vi "XLP80_CAN_MaskBytes_Test01.vi"() -> ()   [LabVIEW 2021]
uses:
  XLP80_FGlob/1886_FGlob_TDefs_Enum_FGlobItems.ctl
  XLP80_Globals/Globals_Settings_XLP80.vi
panel:
  out "Data OUT":u8[](array[numeric])=[0, 7, 255, 248, 0, 24, 0, 0] format="%.0x"
  out "Boolean array Out":bool[](array[boolean])=[FALSE, FALSE, FALSE, FALSE, FALSE, FALSE, FALSE, FALSE, TRUE, TRUE, TRUE, FALSE, FALSE, FALSE, FALSE, FALSE, TRUE, TRUE, TRUE, TRUE, TRUE, TRUE, TRUE, TRUE, FALSE, FALSE, FALSE, TRUE, TRUE, TRUE, TRUE, TRUE, FALSE, FALSE, FALSE, FALSE, FALSE, FALSE, FALSE, FALSE, FALSE, FALSE, FALSE, TRUE, TRUE, FALSE, FALSE, FALSE, FALSE, FALSE, FALSE, FALSE, FALSE, FALSE, FALSE, FALSE, FALSE, FALSE, FALSE, FALSE, FALSE, FALSE, FALSE, FALSE]
  in  "AO Values IN 2":dbl[](array[numeric])=[65535.0, 3.0] format="%.6f"
  in  "Signal Name Write 2":string[](array[string])=["Signal1", "Signal2"]
  out "err out":errorcluster caption="error"
  out "AI Values OUT":dbl[](array[numeric])=[33882.882] format="%.6f"
  in  "stop":bool
  in  "PEAK CANData Read":T1(array[cluster])=[{"ID"=1281, "MSG type"=enum."STD", "LEN"=8, "DATA"=[0, 0, 0, 0, 2, 3, 5, 2]}] {"DATA" format="%.0x"; "ID" format="%.0x"}
  in  "AO Values IN":dbl[](array[numeric])=[1.2, 2.2, 15.0, 14.0] format="%.6f"
  out "CANData Write":T1(array[cluster])=[{"ID"=2047, "MSG type"=enum."STD", "LEN"=8, "DATA"=[0, 7, 255, 248, 0, 24, 0, 0]}] {"DATA" format="%.0x"; "ID" format="%.0x"}
  in  "DBC":path=path "G:/07_GLOBE/00_git/XLP80/02_Documentation/Daten Albert_10-08-2022/TestDBC.dbc"
  in  "Signal Name Write":string[](array[string])=["C07_BAT_s_Max_Cell_Voltage", "C07_BAT_s_Min_Cell_Voltage", "C07_BAT_s_Max_Cell_Temperature", "C07_BAT_s_Min_Cell_Temperature"]
  in  "Signal Name Read":string[](array[string])=["C07_BAT_s_Battery_Voltage"]
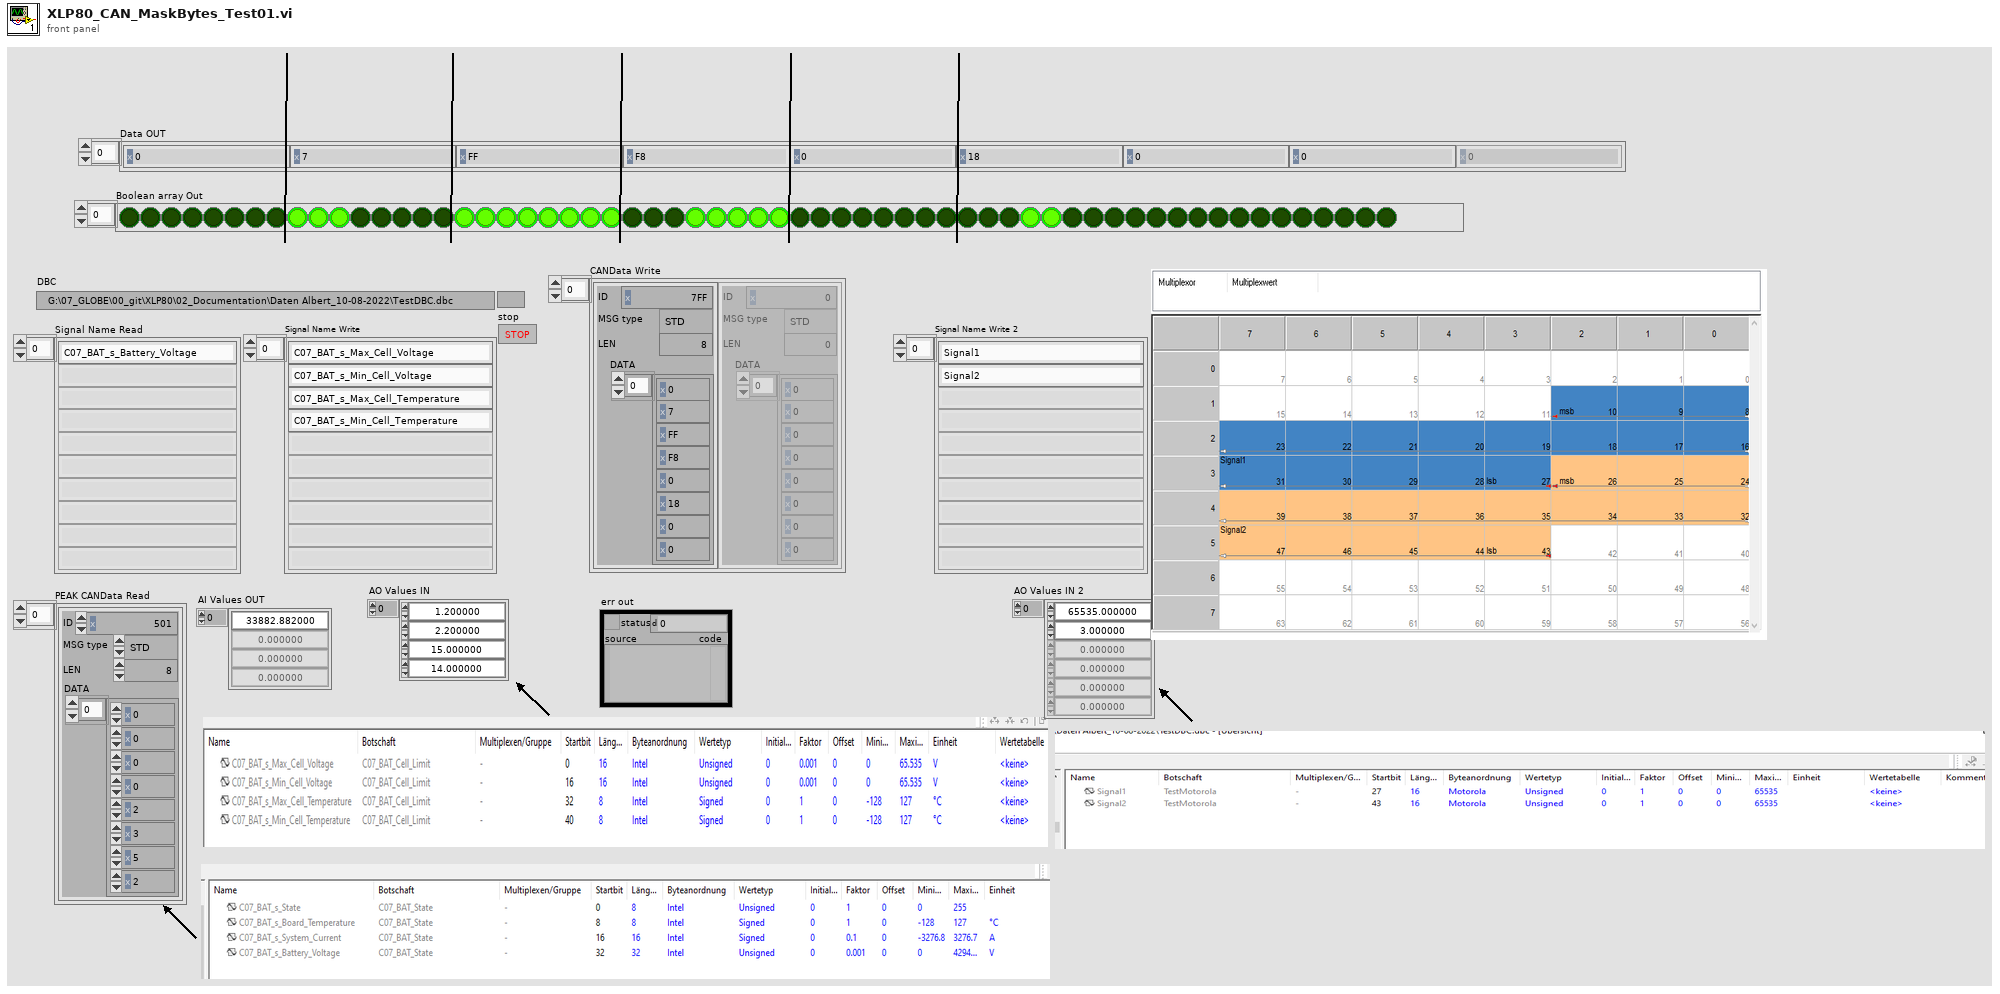
[diagram p1: front panel]
types:
  T1 = cluster{"ID":u32, "MSG type":enum8{"STD", "RTR", "XTD", "XTD RTR", "STATUS"}, "LEN":i8, "DATA":u8[]}[]
  T2 = typedef "1886_FGlob_TDefs_Enum_FGlobItems.ctl" = enum16{"Put one", "Put all", "Recall one", "Recall all"}
  T3 = cluster{"DBC":path, "Signal Name Read":string[], "Signal Name Write 2":string[]}
  T4 = typedef "PCANBasic.lvlib/CAN MSG Cluster.ctl" = cluster{"ID":u32, "MSG type":enum8{"STD", "RTR", "XTD", "XTD RTR", "STATUS"}, "LEN":i8, "DATA":u8[]}
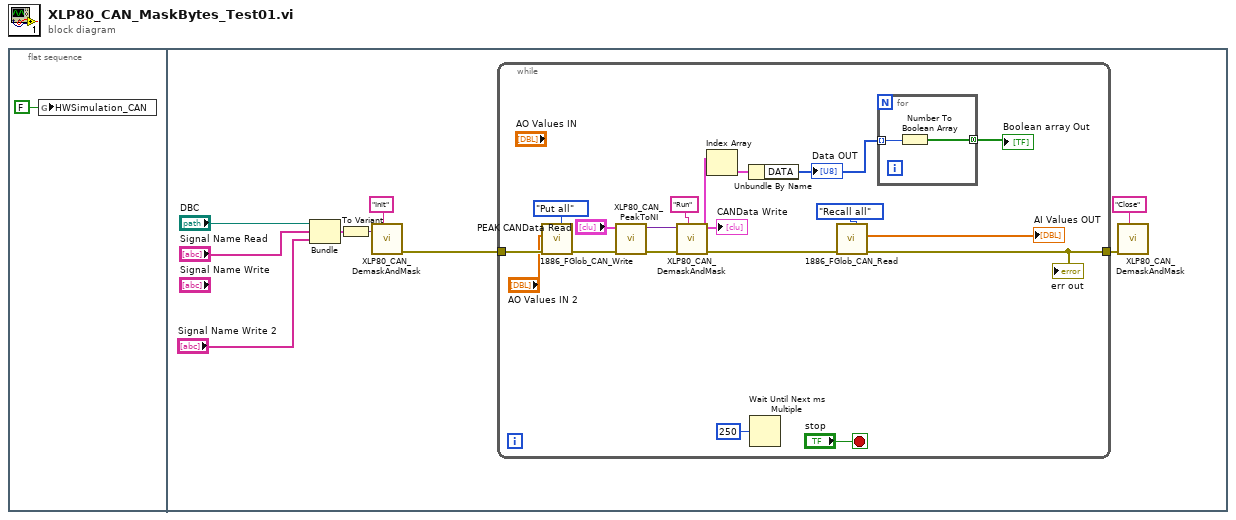
[diagram p0: block diagram]
diagram:
  n1 = flat-sequence {
    frame #0 {
      n2 = global write "Globals_Settings_XLP80.vi" "HWSimulation_CAN"(FALSE ("HWSimulation_CAN")) -> ()
    }
    frame #1 {
      n3 = Bundle("DBC"="DBC", "Signal Name Read"="Signal Name Read", "Signal Name Write 2"="Signal Name Write 2") -> (w10:T3)  [unwired: 1 in]
      n4 = To Variant(anything=w10) -> (Variant=w7:variant)
      n5 = call "XLP80_CAN_DemaskAndMask.vi"("Function"="Init", "Variant"=w7) -> ("error out"=w3:errorcluster)  [unwired: 8 in, 1 out]
      n6 = while {
        tunnel: w3 -> [w26]
        tunnel: [w18] -> w4
        stop <- "stop" stop-if-true
        n7 = call "1886_FGlob_CAN_Write.vi"("Function (Recall One)"=1886_FGlob_TDefs_Enum_FGlobItems."Put all", "AO Values IN"="AO Values IN 2") -> ()  [unwired: 7 in, 3 out]
        n8 = call "XLP80_CAN_PeakToNI.vi"("error in"=w26, "PEAK CANData Read"="PEAK CANData Read") -> ("error out"=w25:errorcluster, "NI Data OUT"=w24:variant)  [unwired: 8 in]
        n9 = call "XLP80_CAN_DemaskAndMask.vi"("Function"="Run", "err in"=w25, "Variant"=w24) -> ("error out"=w19:errorcluster, "CANData Write"=w14:T4[])  [unwired: 7 in]
        "CANData Write" <- w14
        n10 = Index Array(array=w14) -> (element=w13:T4)  [unwired: 1 in]
        n11 = Unbundle By Name(w13) -> ("DATA"=w12:u8[])
        "Data OUT" <- w12
        n12 = Wait Until Next ms Multiple(millisecond multiple=u32 250) -> ()  [unwired: 1 out]
        n13 = call "1886_FGlob_CAN_Read.vi"("Function (Recall One)"=1886_FGlob_TDefs_Enum_FGlobItems."Recall all", "err in"=w19) -> ("err out"=w18:errorcluster, "AI Values OUT"=→"AI Values OUT":dbl[])  [unwired: 7 in, 1 out]
        "err out" <- w18
        n14 = for {
          tunnel: w12 -> [w29] mode=indexing
          tunnel: [w28] -> w11 mode=concatenating
          n15 = Number To Boolean Array(number=w29) -> (Boolean array=w28:bool[])
        }
        "Boolean array Out" <- w11
      }
      n16 = call "XLP80_CAN_DemaskAndMask.vi"("Function"="Close", "err in"=w4) -> ()  [unwired: 8 in, 2 out]
    }
  }
